vi "demo_.NET (Core) 8 Improvements in 2026 Q1.vi"(11 "Stop Demo":refnum<user-event>) -> ()   [LabVIEW 2020]
panel:
  # "LabVIEW 2026 Q1 - .NET (Core) 8.0 Improvements\n\n- Support for probes on .NET (Core) 8.0 reference wires\n- Support for .NET Core APIs which get or set arrays of class references\n- Support for .NET Object to Variant, Variant to .NET Object,\n   To More Generic Class, and To More Specific Class functions"
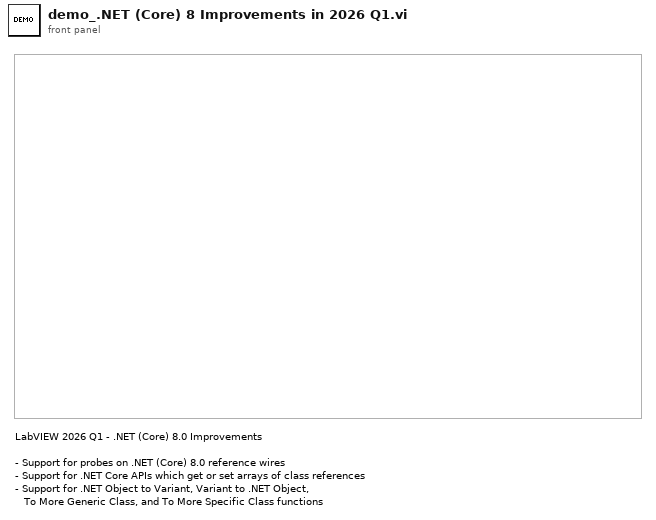
[diagram p1: front panel]
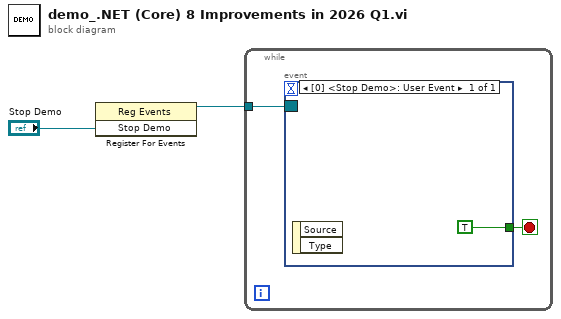
[diagram p0: block diagram]
diagram:
  n1 = register-events("Stop Demo") -> (reference out=w1:refnum<event-registration>)  [unwired: 2 in, 1 out]
  n2 = while {
    tunnel: w1 -> [w4]
    stop <- w3 stop-if-true
    n3 = event shown="[0] <Stop Demo>: User Event" {
      selector: w4 -> [_]
      dyn-events: _ -> [_]
      timeout: _ -> [_]
      tunnel: [TRUE] -> w3
      event User Event {
        n4 = event-data() -> ()  [unwired: 1 in, 2 out]
      }
    }
  }
